vi "Update Method Getter.vi"(7 "RPC Method Name":string, 8 "error in (no error)":errorcluster, 10 "Request Metadata Name":string, 11 "Server class in":refnum<vi>) -> (0 "error out":errorcluster, 3 "Server class out":refnum<vi>)   [LabVIEW 2019, in "gRPC Scripting Tools.lvlib"]
uses:
  gRPC Scripting Tools.lvlib
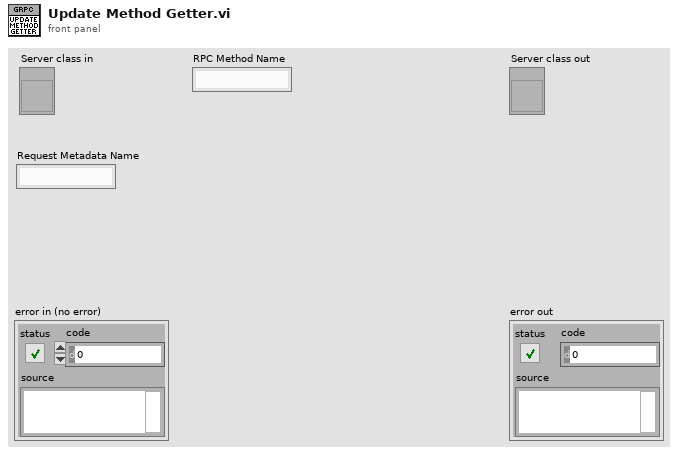
[diagram p1: front panel]
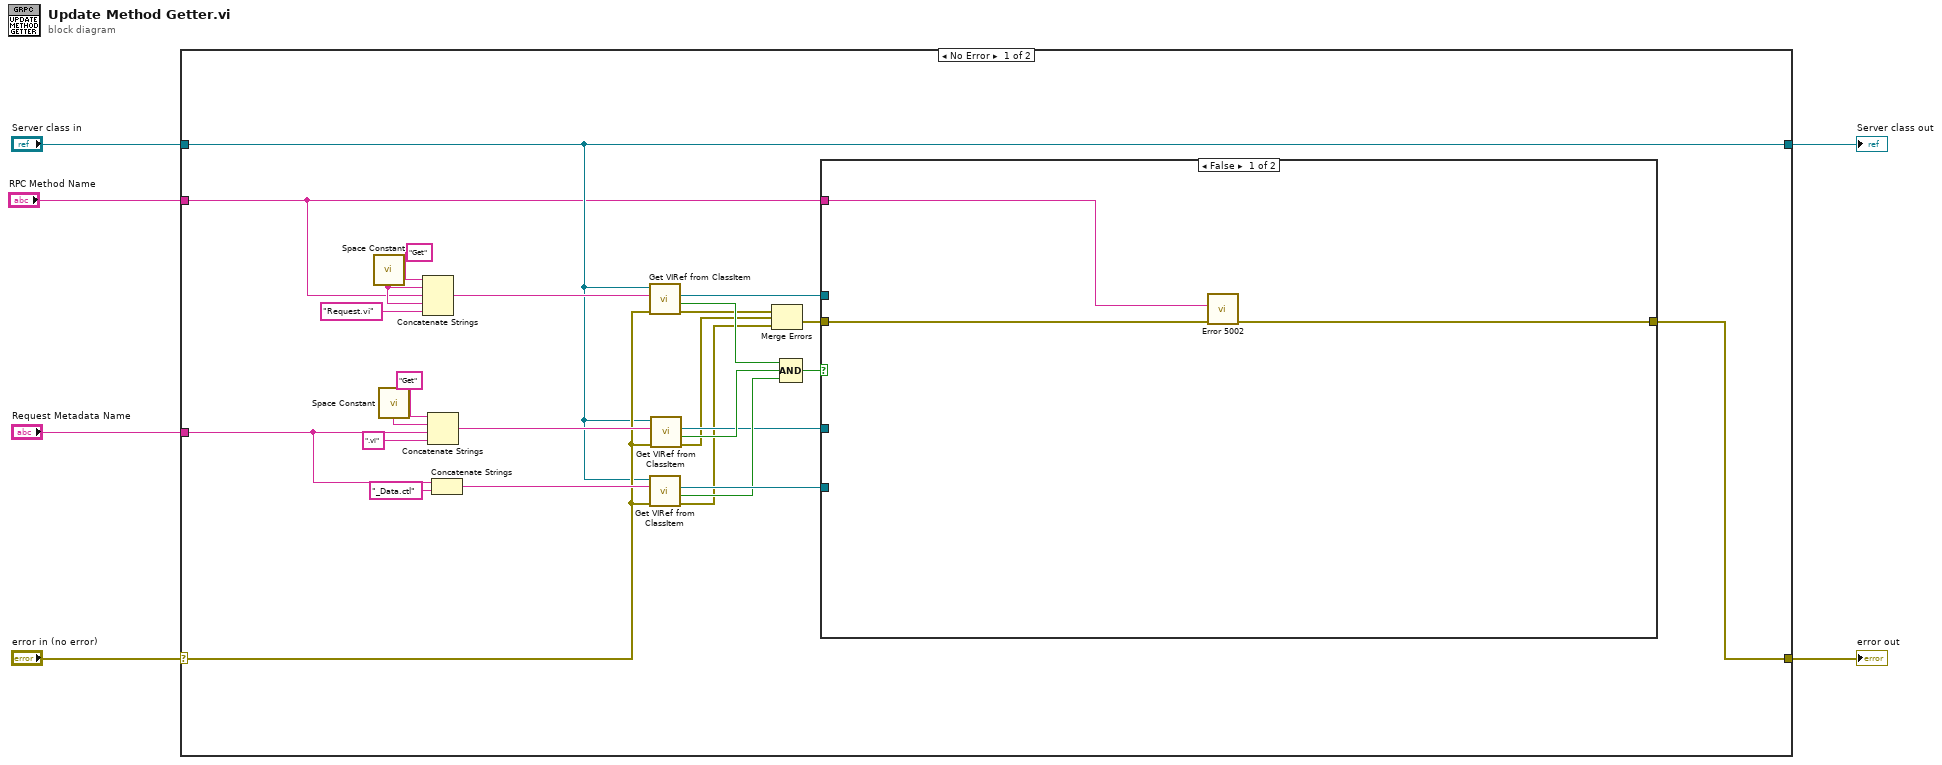
[diagram p0: block diagram]
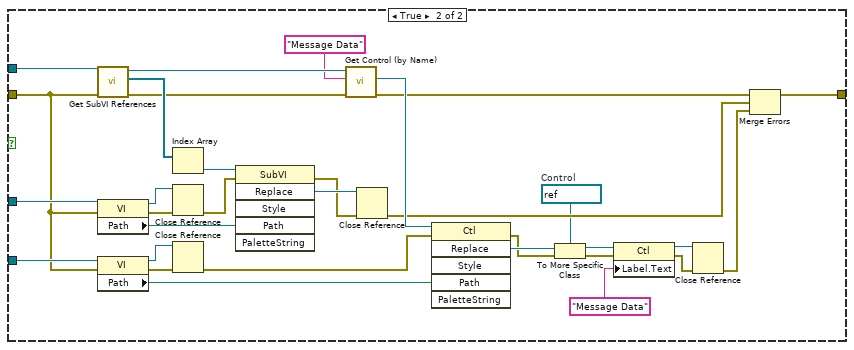
[diagram p2: hidden frame]
diagram:
  n1 = case shown="No Error" "error in (no error)" {
    selector: "error in (no error)" -> [w14 w69]
    tunnel: "Server class in" -> [w8 w68]
    tunnel: "Request Metadata Name" -> [w25 _]
    tunnel: "RPC Method Name" -> [w7 _]
    tunnel: [w9 w69] -> w2
    tunnel: [w8 w68] -> w1
    frame No Error {
      n2 = call <vilib>:"Space Constant.vi"() -> ("String"=w16:string)
      n3 = call <vilib>:"Space Constant.vi"() -> ("String"=w18:string)
      n4 = Concatenate Strings("Get" ("string"), w16, w7, w16, "Request.vi" ("string")) -> (w22:string)
      n5 = Concatenate Strings("Get" ("string"), w18, w25, ".vi" ("string")) -> (w21:string)
      n6 = Concatenate Strings(w25, "_Data.ctl" ("string")) -> (w27:string)
      n7 = call "Get VIRef from ClassItem.vi"("error in (no error)"=w14, "Item Name"=w22, "LVClassLibrary in"=w8) -> ("error out"=w13:errorcluster, "Found ?"=w28:bool, "VIref out"=w23:refnum<vi>)  [unwired: 5 in, 1 out]
      n8 = call "Get VIRef from ClassItem.vi"("error in (no error)"=w14, "Item Name"=w27, "LVClassLibrary in"=w8) -> ("error out"=w10:errorcluster, "Found ?"=w30:bool, "VIref out"=w32:refnum<vi>)  [unwired: 5 in, 1 out]
      n9 = call "Get VIRef from ClassItem.vi"("error in (no error)"=w14, "Item Name"=w21, "LVClassLibrary in"=w8) -> ("error out"=w11:errorcluster, "Found ?"=w29:bool, "VIref out"=w24:refnum<vi>)  [unwired: 5 in, 1 out]
      n10 = Merge Errors(w13, w11, w10) -> (w12:errorcluster)
      n11 = Compound Arithmetic op=AND(w28, w29, w30) -> (w31:bool)
      n12 = case shown="False" w31 {
        tunnel: w23 -> [_ w65]
        tunnel: w24 -> [_ w64]
        tunnel: w32 -> [_ w60]
        tunnel: w12 -> [w35 w54]
        tunnel: [w34 w36] -> w9
        tunnel: w7 -> [w33 _]
        frame False {
          n13 = call "Error 5002.vi"("error in (no error)"=w35, "Method Name"=w33) -> ("error out"=w34:errorcluster)  [unwired: 9 in]
        }
        frame True {
          w43 = refnum<vi> refnum  # Control
          n14 = call "Get SubVI References.vi"("error in (no error)"=w54, "Owner vi in"=w65) -> ("error out"=w55:errorcluster, "SubVI refs"=w67:refnum<vi>[], "Owner vi out"=w58:refnum<vi>)  [unwired: 7 in]
          n15 = property class="VI"(reference=w64, error in=w54) -> (reference out=w50:refnum<vi>, error out=w51:errorcluster, "Path"=w63:path)
          n16 = property class="VI"(reference=w60, error in=w54) -> (reference out=w48:refnum<vi>, error out=w49:errorcluster, "Path"=w59:path)
          n17 = Index Array(array=w67) -> (element=w66:refnum<vi>)  [unwired: 1 in]
          n18 = Close Reference(reference=w50, error in (no error)=w51) -> (error out=w46:errorcluster)
          n19 = Close Reference(reference=w48, error in (no error)=w49) -> (error out=w47:errorcluster)
          n20 = invoke class="SubVI" method="Replace"(reference=w66, error in=w46, "Path"=w63) -> (error out=w61:errorcluster, "Replace"=w62:refnum<vi>)  [unwired: 3 in, 4 out]
          n21 = call "Get Control (by Name).vi"("error in (no error)"=w55, "Control Label"="Message Data" ("Constant Label"), "Owner VI in"=w58) -> ("error out"=w53:errorcluster, "Control Refnum"=w56:refnum<vi>)  [unwired: 5 in, 2 out]
          n22 = Close Reference(reference=w62, error in (no error)=w61) -> (error out=w52:errorcluster)
          n23 = invoke class="Ctl" method="Replace"(reference=w56, error in=w47, "Path"=w59) -> (error out=w44:errorcluster, "Replace"=w45:refnum<vi>)  [unwired: 3 in, 4 out]
          n24 = To More Specific Class(target class=w43, reference=w45, error in=w44) -> (specific class reference=w41:refnum<vi>, error out=w42:errorcluster)
          n25 = property class="Ctl"(reference=w41, error in=w42, "Label.Text"="Message Data") -> (reference out=w38:refnum<vi>, error out=w39:errorcluster)
          n26 = Close Reference(reference=w38, error in (no error)=w39) -> (error out=w37:errorcluster)
          n27 = Merge Errors(w53, w52, w37) -> (w36:errorcluster)
        }
      }
    }
    frame Error {
    }
  }
  "Server class out" <- w1
  "error out" <- w2
